vi "Destroy User Events.vi"(11 "UI Actor in":refnum<class "UI Actor.lvclass">) -> (3 "UI Actor out":refnum<class "UI Actor.lvclass">)   [LabVIEW 2019, in "UI Actor.lvlib" / "UI Actor.lvclass"]
uses:
  UI Actor.lvclass
  UI Actor.lvclass/UI Actor.ctl
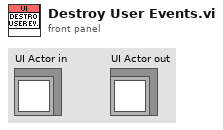
[diagram p1: front panel]
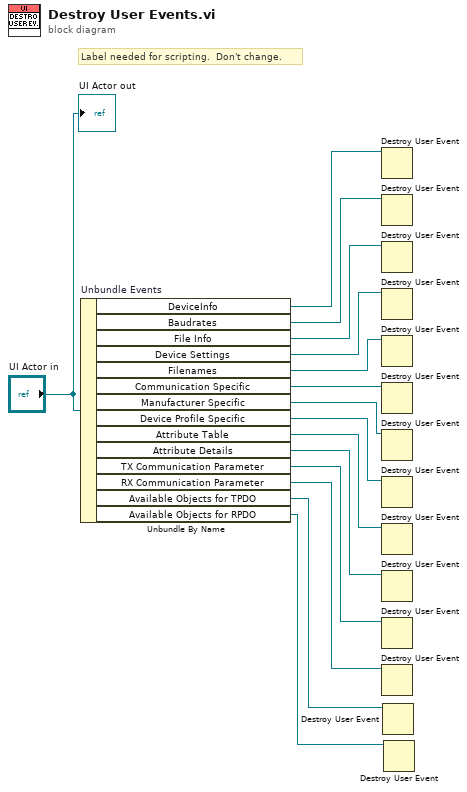
[diagram p0: block diagram]
diagram:
  # "Label needed for scripting.  Don't change."
  n1 = Unbundle By Name "Unbundle Events"("UI Actor in") -> ("DeviceInfo"=w15:refnum<user-event>, "Baudrates"=w13:refnum<user-event>, "File Info"=w12:refnum<user-event>, "Device Settings"=w11:refnum<user-event>, "Filenames"=w10:refnum<user-event>, "Communication Specific"=w9:refnum<user-event>, "Manufacturer Specific"=w8:refnum<user-event>, "Device Profile Specific"=w7:refnum<user-event>, "Attribute Table"=w6:refnum<user-event>, "Attribute Details"=w5:refnum<user-event>, "TX Communication Parameter"=w4:refnum<user-event>, "RX Communication Parameter"=w3:refnum<user-event>, "Available Objects for TPDO"=w2:refnum<user-event>, "Available Objects for RPDO"=w1:refnum<user-event>)
  n2 = Destroy User Event(user event=w15) -> ()  [unwired: 1 in, 1 out]
  n3 = Destroy User Event(user event=w13) -> ()  [unwired: 1 in, 1 out]
  n4 = Destroy User Event(user event=w12) -> ()  [unwired: 1 in, 1 out]
  n5 = Destroy User Event(user event=w11) -> ()  [unwired: 1 in, 1 out]
  n6 = Destroy User Event(user event=w10) -> ()  [unwired: 1 in, 1 out]
  n7 = Destroy User Event(user event=w9) -> ()  [unwired: 1 in, 1 out]
  n8 = Destroy User Event(user event=w8) -> ()  [unwired: 1 in, 1 out]
  n9 = Destroy User Event(user event=w7) -> ()  [unwired: 1 in, 1 out]
  n10 = Destroy User Event(user event=w6) -> ()  [unwired: 1 in, 1 out]
  n11 = Destroy User Event(user event=w5) -> ()  [unwired: 1 in, 1 out]
  n12 = Destroy User Event(user event=w4) -> ()  [unwired: 1 in, 1 out]
  n13 = Destroy User Event(user event=w3) -> ()  [unwired: 1 in, 1 out]
  n14 = Destroy User Event(user event=w2) -> ()  [unwired: 1 in, 1 out]
  n15 = Destroy User Event(user event=w1) -> ()  [unwired: 1 in, 1 out]
  "UI Actor out" <- "UI Actor in"
